vi "LJstreamM globals.vi"() -> ()   [LabVIEW 2025]
panel:
  in  "Defaults Open Any":string="LJM_Open_Any.cfg"
  in  "Defaults Config Name":string="LJM_Default_Configs.cfg"
  in  "Graph?":bool[](array[boolean])=[FALSE, FALSE, FALSE, FALSE, FALSE, FALSE, FALSE, FALSE, FALSE, FALSE, FALSE, FALSE, FALSE, FALSE, FALSE, FALSE]
  in  "Graph Buffer":dbl[][](array[numeric]) format="%.3f"
  in  "Working Directory":path
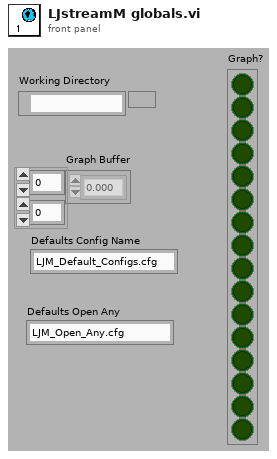
[diagram p1: front panel]
diagram:
